vi "UDP Dispatcher.vi"(0 "UDP port (0)":u16, 5 "use any port (F)":bool, 11 "error in":errorcluster) -> (15 "error out":errorcluster)   [LabVIEW 2015, in "TLB` Template.lvlib" / "AMC.lvlib"]
doc: "TLB Prime - Application Template 1.3.0.24\nNorm Kirchner, NI Systems Engineering - NI\nCopyright (c) 2014, NI"
uses:
  AMC.lvlib
  Dispatcher State Variables.ctl
  FG Dispatcher Status Action.ctl
  Read Termination Message.vi
  Map String.vi
  <vilib>/Utility/error.llb/Clear Errors.vi
  Get Case Matching.vi
  Queue Registry.vi
  Globals.vi
  Tools_KeyedArray.lvlib
panel:
  in  "init complete":refnum<notifier>
  out "dispatcher error":errorcluster
  out "source process":string
  out "source host":string
  in  "stop":bool
  out "message string":string
  out "status":string
  # "Receive"
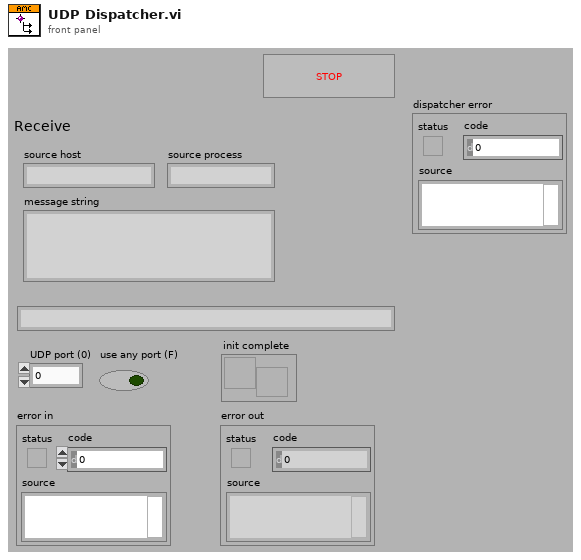
[diagram p1: front panel]
types:
  T1 = typedef "TLB` Template.lvlib/AMC.lvlib/Dispatcher State Variables.ctl" = cluster{"UDP conn ID":refnum<k16>, "UDP port":u16}
  T2 = typedef "TLB` Template.lvlib/AMC.lvlib/Message Queue.ctl" = refnum<queue>
  T3 = typedef "TLB` Template.lvlib/AMC.lvlib/FG Dispatcher Status Action.ctl" = enum16{"Get", "Force Init", "Close"}
  T4 = typedef "TLB` Template.lvlib/AMC.lvlib/Message.ctl" = cluster{"name":string, "value":string, "attributes":T5, "receiver host":string, "receiver process":string, "source host":string, "source process":string, "priority message":bool, "acknowledge message":bool}
  T5 = typedef "TLB` Template.lvlib/Tools_KeyedArray.lvlib/KeyedArray.ctl" = cluster{"keys":string[], "values":string[]}
  T6 = typedef "TLB` Template.lvlib/AMC.lvlib/Queue Registry Properties.ctl" = cluster{"Name":string}
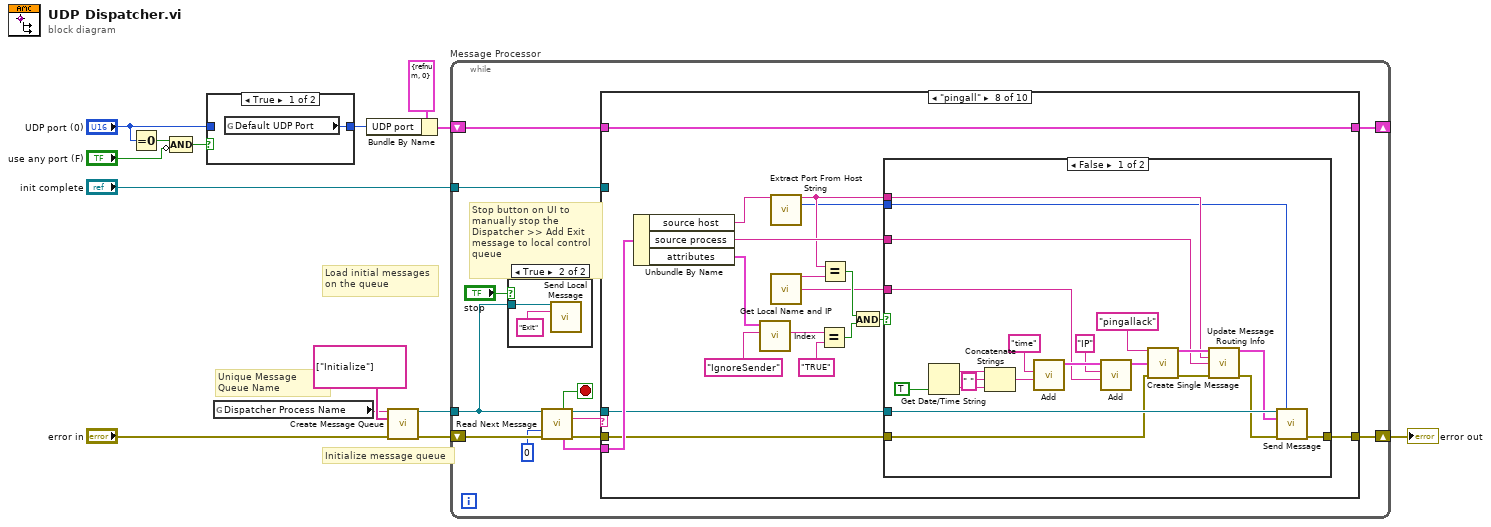
[diagram p0: block diagram]
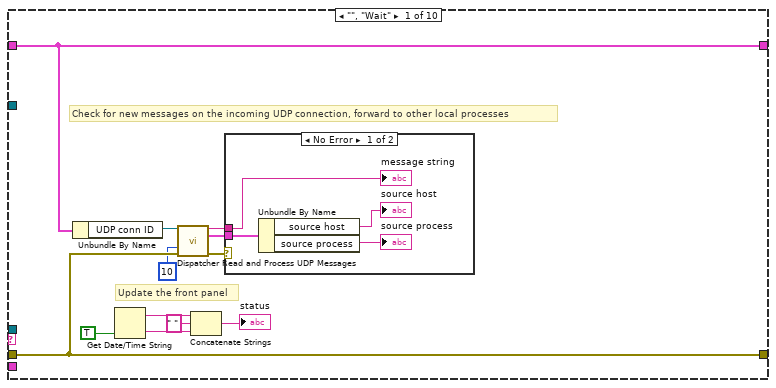
[diagram p4: hidden frame]
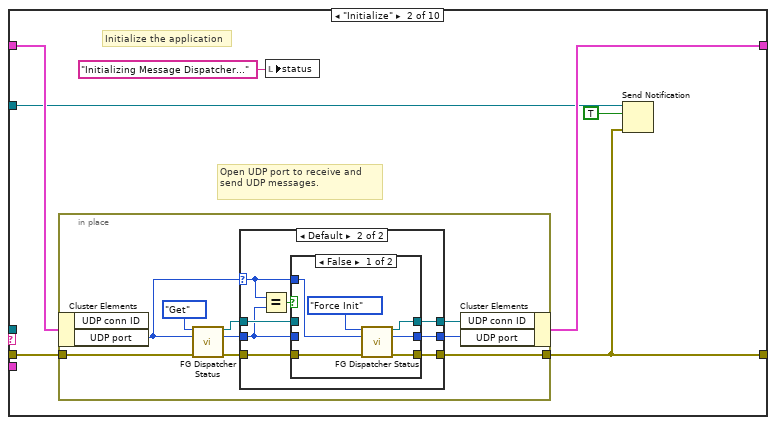
[diagram p6: hidden frame]
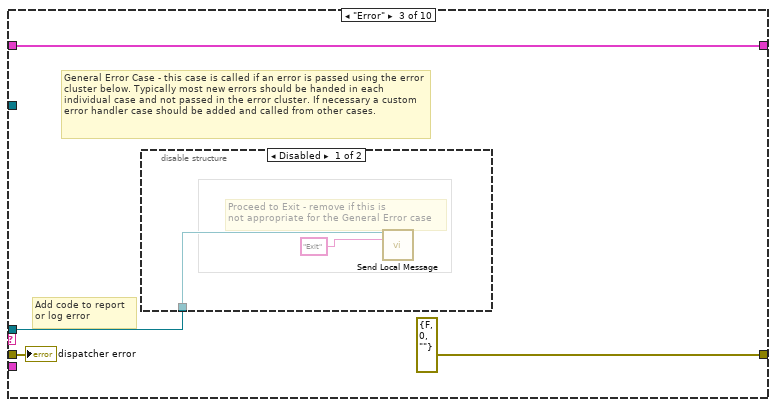
[diagram p9: hidden frame]
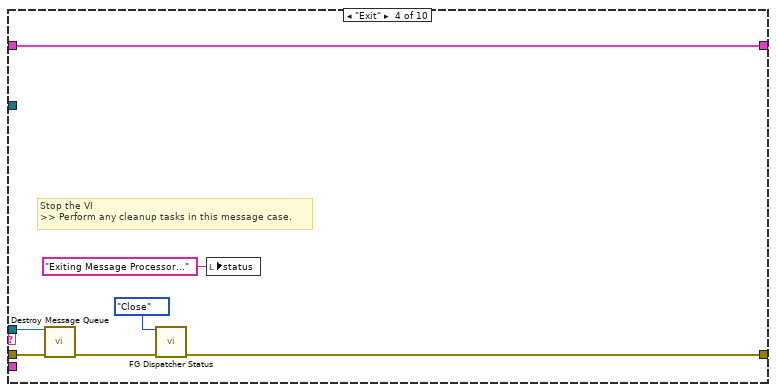
[diagram p11: hidden frame]
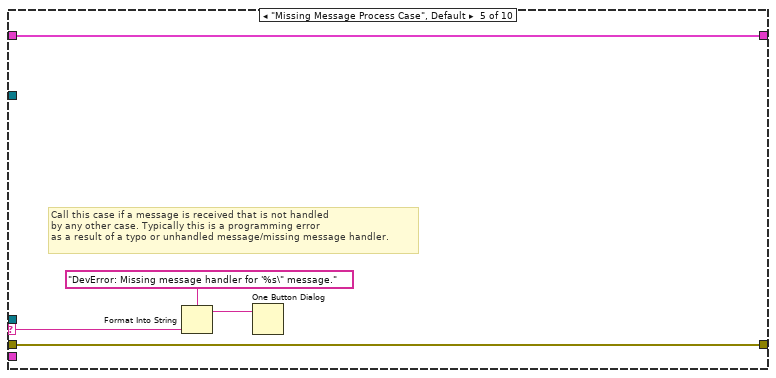
[diagram p12: hidden frame]
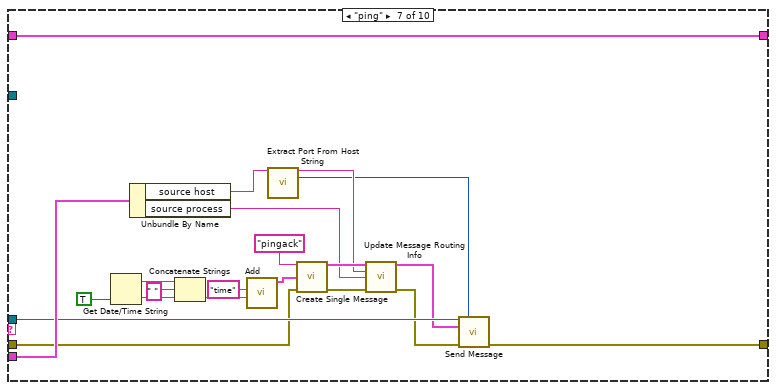
[diagram p14: hidden frame]
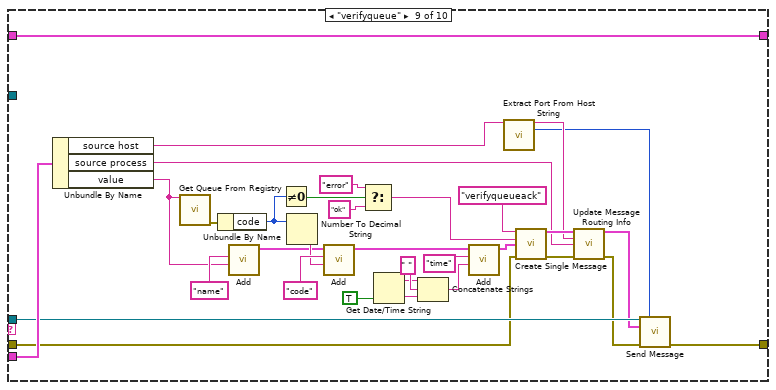
[diagram p16: hidden frame]
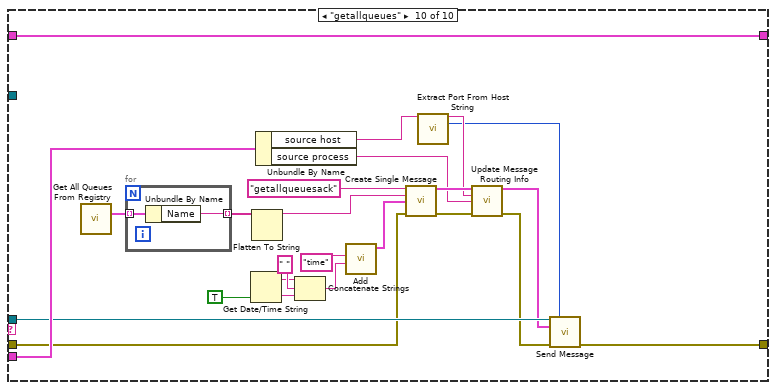
[diagram p17: hidden frame]
diagram:
  # "Initialize message queue"
  # "Unique Message Queue Name"
  # "Load initial messages\non the queue"
  n1 = Equal To 0?(x="UDP port (0)") -> (x = 0?=w4:bool)
  n2 = Compound Arithmetic op=AND(w4, invert "use any port (F)") -> (w2:bool)
  n3 = case shown="True" w2 {
    tunnel: [w15 w16] -> w5
    tunnel: "UDP port (0)" -> [_ w16]
    frame True {
      n4 = global read "Globals.vi" "Default UDP Port"() -> (w15:u16)
    }
    frame False {
    }
  }
  n5 = global read "Globals.vi" "Dispatcher Process Name"() -> (w11:string)
  n6 = Bundle By Name(cluster=T1 {"UDP conn ID"=refnum, "UDP port"=0} ("state variables"), "UDP port"=w5) -> (w9:T1)
  n7 = call "Create Message Queue.vi"("message queue name"=w11, "initial message names"=string[] ["Initialize"], "error in"="error in") -> ("message queue out"=w14:T2, "error out"=w13:errorcluster)  [unwired: 11 in]
  n8 = while "Message Processor" {
    shift-left: w13 -> [w25]
    shift-right: [w26] -> w7
    tunnel: w14 -> [w21]
    shift-left: w9 -> [w29]
    shift-right: [w20] -> _
    tunnel: "init complete" -> [w18]
    stop <- w23 stop-if-true
    # "Stop button on UI to\nmanually stop the\nDispatcher >> Add Exit\nmessage to local control\nqueue"
    n9 = case shown="True" "stop" {
      tunnel: w21 -> [_ w30]
      frame False {
      }
      frame True {
        n10 = call "Send Local Message.vi"("message queue in"=w30, "message name"="Exit") -> ()  [unwired: 11 in, 3 out]
      }
    }
    n11 = call "Read Next Message.vi"("message queue in"=w21, "timeout (1 ms)"=0 ("timeout (1ms)"), "error in"=w25) -> ("exit process?"=w23:bool, "message queue out"=w28:T2, "message name"=w24:string, "message"=w19:T4, "error out"=w27:errorcluster)  [unwired: 5 in, 3 out]
    n12 = case shown="\"pingall\"" w24 {
      selector: w24 -> [_ _ _ _ w99 _ _ _ _ _]
      tunnel: w29 -> [w38 w53 w87 w94 w101 w103 w124 w142 w197 w221]
      tunnel: w28 -> [_ _ w85 w95 _ _ w113 w129 w174 w209]
      tunnel: w27 -> [w34 w51 w84 w96 w100 w102 w109 w131 w170 w202]
      tunnel: [w34 w49 errorcluster {"status"=FALSE, "code"=0, "source"=""} ("error out") w90 w100 w102 w116 w130 w178 w212] -> w26
      tunnel: [w38 w52 w87 w94 w101 w103 w124 w142 w197 w221] -> w20
      tunnel: w19 -> [_ _ _ _ _ _ w123 w141 w196 w220]
      tunnel: w18 -> [_ w50 _ _ _ _ _ _ _ _]
      frame "", "Wait" {
        # "Check for new messages on the incoming UDP connection, forward to other local processes"
        # "Update the front panel"
        n13 = Unbundle By Name(w38) -> ("UDP conn ID"=w36:refnum<k16>)
        n14 = Get Date/Time String(want seconds? (F)=TRUE) -> (date string=w43:string, time string=w42:string)  [unwired: 2 out]
        n15 = call "Dispatcher Read and Process UDP Messages.vi"("UDP conn ID"=w36, "timeout (10 ms)"=10, "error in"=w34) -> ("message string"=w37:string, "message"=w32:T4, "error out"=w35:errorcluster)  [unwired: 10 in]
        n16 = Concatenate Strings(w43, " " ("string"), w42) -> (→"status":string)
        n17 = case shown="No Error" w35 {
          tunnel: w37 -> [w47 _]
          tunnel: w32 -> [w46 _]
          frame No Error {
            n18 = Unbundle By Name(w46) -> ("source host"=→"source host":string, "source process"=→"source process":string)
            "message string" <- w47
          }
          frame Error {
          }
        }
      }
      frame "Initialize" {
        # "Open UDP port to receive and send UDP messages."
        # "Initialize the application"
        n19 = in-place {
          in-place-border: w51 -> [w62]
          in-place-border: [w55] -> w49
          n20 = in-place-cluster #1(w53) -> ("UDP port"=w61:u16)  [unwired: 1 out]
          n21 = call "FG Dispatcher Status.vi"("action (Get)"=FG_Dispatcher_Status_Action."Get", "UDP port in (0)"=w61, "error in"=w62) -> ("UDP connection ID"=w58:refnum<k16>, "UDP port out"=w60:u16, "error out"=w59:errorcluster)  [unwired: 10 in]
          n22 = case shown="Default" w61 {
            selector: w61 -> [_ w67]
            tunnel: w60 -> [w65 w69]
            tunnel: w59 -> [w64 w73]
            tunnel: w58 -> [w66 w71]
            tunnel: [w66 w70] -> w57
            tunnel: [w65 w68] -> w56
            tunnel: [w64 w72] -> w55
            frame 0 {
            }
            frame Default {
              n23 = Equal?(x=w67, y=w69) -> (x = y?=w74:bool)
              n24 = case shown="False" w74 {
                tunnel: w73 -> [w78 w83]
                tunnel: [w77 w83] -> w72
                tunnel: w71 -> [_ w82]
                tunnel: [w79 w82] -> w70
                tunnel: w69 -> [_ w81]
                tunnel: [w75 w81] -> w68
                tunnel: w67 -> [w76 _]
                frame False {
                  n25 = call "FG Dispatcher Status.vi"("action (Get)"=FG_Dispatcher_Status_Action."Force Init", "UDP port in (0)"=w76, "error in"=w78) -> ("UDP connection ID"=w79:refnum<k16>, "UDP port out"=w75:u16, "error out"=w77:errorcluster)  [unwired: 10 in]
                }
                frame True {
                }
              }
            }
          }
          n26 = in-place-cluster #1("UDP conn ID"=w57, "UDP port"=w56) -> (w52:T1)
        }
        n27 = local write "status"("Initializing Message Dispatcher..." ("message")) -> ()
        n28 = Send Notification(notification=TRUE, notifier=w50, error in (no error)=w49) -> ()  [unwired: 2 out]
      }
      frame "Error" {
        # "Add code to report\nor log error"
        # "General Error Case - this case is called if an error is passed using the error cluster below. Typically most new errors should be handed in each individual case and not passed in the error cluster. If necessary a custom error handler case should be added and called from other cases."
        n29 = disable-structure shown="Disabled" {
          disable-tunnel: w85 -> [w89 _]
          frame Disabled {
            # "Proceed to Exit - remove if this is\nnot appropriate for the General Error case"
            n30 = call "Send Local Message.vi"("message queue in"=w89, "message name"="Exit") -> ()  [unwired: 11 in, 3 out]
          }
          frame Enabled {
          }
        }
        "dispatcher error" <- w84
      }
      frame "Exit" {
        # "Stop the VI\n>> Perform any cleanup tasks in this message case."
        n31 = call "Destroy Message Queue.vi"("message queue in"=w95, "error in"=w96) -> ("error out"=w91:errorcluster)  [unwired: 11 in, 2 out]
        n32 = call "FG Dispatcher Status.vi"("action (Get)"=FG_Dispatcher_Status_Action."Close", "error in"=w91) -> ("error out"=w90:errorcluster)  [unwired: 11 in, 2 out]
        n33 = local write "status"("Exiting Message Processor..." ("button name (\"OK\")")) -> ()
      }
      frame "Missing Message Process Case", Default {
        # "Call this case if a message is received that is not handled \nby any other case. Typically this is a programming error\nas a result of a typo or unhandled message/missing message handler."
        n34 = Format Into String(format string="DevError: Missing message handler for '%s\" message." ("message"), w99) -> (resulting string=w97:string)  [unwired: 2 in, 1 out]
        n35 = One Button Dialog(message=w97) -> ()  [unwired: 2 out]
      }
      frame "**** Message Dispatcher Service Functions ****" {
      }
      frame "ping" {
        n36 = Get Date/Time String(want seconds? (F)=TRUE) -> (date string=w122:string, time string=w121:string)  [unwired: 2 out]
        n37 = Unbundle By Name(w123) -> ("source host"=w106:string, "source process"=w111:string)
        n38 = Concatenate Strings(w122, " ", w121) -> (w119:string)
        n39 = call "Add.vi"("value"=w119, "key"="time") -> ("array out"=w114:T5)  [unwired: 2 in, 3 out]
        n40 = call "Extract Port From Host String.vi"("host in"=w106) -> ("host out"=w105:string, "port"=w104:u16)  [unwired: 12 in, 1 out]
        n41 = call "Create Single Message.vi"("name"="pingack" ("Name"), "attributes"=w114, "error in"=w109) -> ("message"=w112:T4, "error out"=w110:errorcluster)  [unwired: 11 in]
        n42 = call "Update Message Routing Info.vi"("message"=w112, "receiver host (\"\")"=w105, "receiver process (\"\")"=w111, "error in"=w110) -> ("message"=w108:T4, "error out"=w107:errorcluster)  [unwired: 10 in]
        n43 = call "Send Message.vi"("message queue in"=w113, "receiver port (0)"=w104, "message"=w108, "error in"=w107) -> ("error out"=w116:errorcluster)  [unwired: 9 in, 2 out]
      }
      frame "pingall" {
        n44 = Unbundle By Name(w141) -> ("source host"=w127:string, "source process"=w136:string, "attributes"=w140:T5)
        n45 = call "Index.vi"("key"="IgnoreSender", "array in"=w140) -> ("value"=w138:string)  [unwired: 2 in, 3 out]
        n46 = call "Extract Port From Host String.vi"("host in"=w127) -> ("host out"=w126:string, "port"=w125:u16)  [unwired: 12 in, 1 out]
        n47 = call "Get Local Name and IP.vi"() -> ("name"=w132:string, "IP address"=w128:string)  [unwired: 12 in, 2 out]
        n48 = Equal?(x=w138, y="TRUE" ("x")) -> (x = y?=w135:bool)
        n49 = Equal?(x=w126, y=w132) -> (x = y?=w134:bool)
        n50 = And(x=w134, y=w135) -> (x .and. y?=w133:bool)
        n51 = case shown="False" w133 {
          tunnel: w126 -> [w149 _]
          tunnel: w136 -> [w148 _]
          tunnel: w128 -> [w155 _]
          tunnel: w131 -> [w146 w164]
          tunnel: [w154 w164] -> w130
          tunnel: w129 -> [w151 _]
          tunnel: w125 -> [w143 _]
          frame False {
            n52 = Get Date/Time String(want seconds? (F)=TRUE) -> (date string=w163:string, time string=w162:string)  [unwired: 2 out]
            n53 = Concatenate Strings(w163, " ", w162) -> (w160:string)
            n54 = call "Add.vi"("value"=w160, "key"="time") -> ("array out"=w157:T5)  [unwired: 2 in, 3 out]
            n55 = call "Add.vi"("value"=w155, "key"="IP", "array in"=w157) -> ("array out"=w152:T5)  [unwired: 1 in, 3 out]
            n56 = call "Create Single Message.vi"("name"="pingallack" ("Name"), "attributes"=w152, "error in"=w146) -> ("message"=w150:T4, "error out"=w147:errorcluster)  [unwired: 11 in]
            n57 = call "Update Message Routing Info.vi"("message"=w150, "receiver host (\"\")"=w149, "receiver process (\"\")"=w148, "error in"=w147) -> ("message"=w145:T4, "error out"=w144:errorcluster)  [unwired: 10 in]
            n58 = call "Send Message.vi"("message queue in"=w151, "receiver port (0)"=w143, "message"=w145, "error in"=w144) -> ("error out"=w154:errorcluster)  [unwired: 9 in, 2 out]
          }
          frame True {
            # "Do not respond if the PingAll request was sent by this system."
          }
        }
      }
      frame "verifyqueue" {
        n59 = Unbundle By Name(w196) -> ("source host"=w167:string, "source process"=w171:string, "value"=w180:string)
        n60 = call "Get Queue From Registry.vi"("name"=w180) -> ("error out"=w179:errorcluster)  [unwired: 13 in, 1 out]
        n61 = Unbundle By Name(w179) -> ("code"=w191:i32)
        n62 = call "Add.vi"("value"=w180, "key"="name") -> ("array out"=w193:T5)  [unwired: 2 in, 3 out]
        n63 = Not Equal To 0?(x=w191) -> (x != 0?=w190:bool)
        n64 = Number To Decimal String(number=w191) -> (decimal integer string=w194:string)  [unwired: 1 out]
        n65 = call "Add.vi"("value"=w194, "key"="code", "array in"=w193) -> ("array out"=w181:T5)  [unwired: 1 in, 3 out]
        n66 = Select(t="error", s=w190, f="ok") -> (s? t:f=w176:string)
        n67 = Get Date/Time String(want seconds? (F)=TRUE) -> (date string=w185:string, time string=w184:string)  [unwired: 2 out]
        n68 = Concatenate Strings(w185, " ", w184) -> (w183:string)
        n69 = call "Add.vi"("value"=w183, "key"="time", "array in"=w181) -> ("array out"=w175:T5)  [unwired: 1 in, 3 out]
        n70 = call "Extract Port From Host String.vi"("host in"=w167) -> ("host out"=w166:string, "port"=w165:u16)  [unwired: 12 in, 1 out]
        n71 = call "Create Single Message.vi"("name"="verifyqueueack" ("Name"), "value"=w176, "attributes"=w175, "error in"=w170) -> ("message"=w173:T4, "error out"=w168:errorcluster)  [unwired: 10 in]
        n72 = call "Update Message Routing Info.vi"("message"=w173, "receiver host (\"\")"=w166, "receiver process (\"\")"=w171, "error in"=w168) -> ("message"=w172:T4, "error out"=w169:errorcluster)  [unwired: 10 in]
        n73 = call "Send Message.vi"("message queue in"=w174, "receiver port (0)"=w165, "message"=w172, "error in"=w169) -> ("error out"=w178:errorcluster)  [unwired: 9 in, 2 out]
      }
      frame "getallqueues" {
        n74 = call "Get All Queues From Registry.vi"() -> ("all properties"=w213:T6[])  [unwired: 12 in, 3 out]
        n75 = for {
          tunnel: w213 -> [w223] mode=indexing
          tunnel: [w222] -> w208 mode=indexing
          n76 = Unbundle By Name(w223) -> ("Name"=w222:string)
        }
        n77 = Get Date/Time String(want seconds? (F)=TRUE) -> (date string=w217:string, time string=w216:string)  [unwired: 2 out]
        n78 = Flatten To String(anything=w208) -> (data string=w207:string)  [unwired: 3 in, 2 out]
        n79 = Unbundle By Name(w220) -> ("source host"=w200:string, "source process"=w204:string)
        n80 = Concatenate Strings(w217, " ", w216) -> (w215:string)
        n81 = call "Add.vi"("value"=w215, "key"="time") -> ("array out"=w210:T5)  [unwired: 2 in, 3 out]
        n82 = call "Create Single Message.vi"("name"="getallqueuesack" ("Name"), "value"=w207, "attributes"=w210, "error in"=w202) -> ("message"=w206:T4, "error out"=w203:errorcluster)  [unwired: 10 in]
        n83 = call "Extract Port From Host String.vi"("host in"=w200) -> ("host out"=w199:string, "port"=w198:u16)  [unwired: 12 in, 1 out]
        n84 = call "Update Message Routing Info.vi"("message"=w206, "receiver host (\"\")"=w199, "receiver process (\"\")"=w204, "error in"=w203) -> ("message"=w205:T4, "error out"=w201:errorcluster)  [unwired: 10 in]
        n85 = call "Send Message.vi"("message queue in"=w209, "receiver port (0)"=w198, "message"=w205, "error in"=w201) -> ("error out"=w212:errorcluster)  [unwired: 9 in, 2 out]
      }
    }
  }
  "error out" <- w7
